vi "Configure Device.vi"(8 "error in":errorcluster, 11 "SR3XXX HVPS in":refnum<class "SR3XXX HVPS.lvclass">) -> (0 "error out":errorcluster, 3 "SR3XXX HVPS out":refnum<class "SR3XXX HVPS.lvclass">)   [LabVIEW 2014, in "SR3XXX HVPS.lvclass"]
uses:
  SR3XXX HVPS.lvclass
  <vilib>/Utility/config.llb/NI_LVConfig.lvlib
  reusable/Session APIs/File Access/Config Data/Config Data.lvclass
  <vilib>/Utility/config.llb/Read Key (String).vi
  <vilib>/Utility/config.llb/Read Key (Double).vi
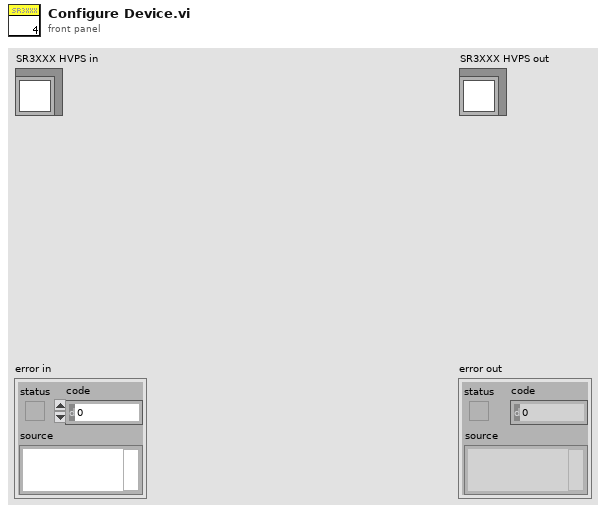
[diagram p1: front panel]
types:
  T1 = typedef "Config Data.lvclass/Config Session.ctl" = refnum<data-value>
  T2 = typedef "NI_LVConfig.lvlib/Config Data RefNum.ctl" = refnum<k1>
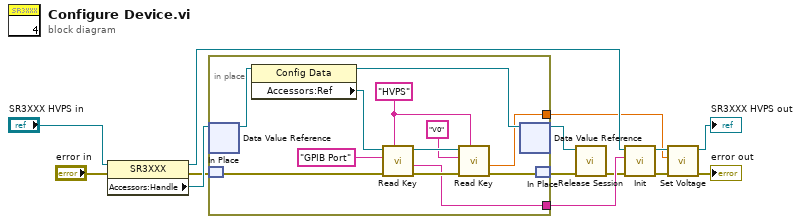
[diagram p0: block diagram]
diagram:
  n1 = property class="SR3XXX"(reference="SR3XXX HVPS in", error in="error in") -> (reference out=w9:refnum<class "SR3XXX HVPS.lvclass">, error out=w11:errorcluster, "Accessors:Handle"=w13:T1)
  n2 = in-place {
    in-place-border: [w16] -> w10
    in-place-border: [w15] -> w6
    w21 = "HVPS" ("section")
    n3 = in-place-dvr #1(w13) -> (w26:refnum<class "Config Data.lvclass">)  [unwired: 1 out]
    n4 = in-place-match #2(w11) -> (w18:errorcluster)
    n5 = property class="Config Data"(reference=w26) -> (reference out=w19:refnum<class "Config Data.lvclass">, "Accessors:Ref"=w25:T2)  [unwired: 1 in, 1 out]
    n6 = call-poly <vilib>:"Read Key.vi"("section"=w21, "error in (no error)"=w18, "key"="GPIB Port" ("section"), "refnum"=w25) -> ("error out"=w23:errorcluster, "value"=w16:string, "refnum out"=w22:T2)  [unwired: 4 in, 1 out]
    n7 = call-poly <vilib>:"Read Key.vi"("section"=w21, "error in (no error)"=w23, "key"="V0", "refnum"=w22) -> ("error out"=w17:errorcluster, "value"=w15:dbl)  [unwired: 4 in, 2 out]
    n8 = in-place-dvr #1(w19) -> (w3:T1)  [unwired: 1 out]
    n9 = in-place-match #2(w17) -> (w2:errorcluster)
  }
  n10 = call "Release Session.vi"("error in"=w2, "Session Handle"=w3) -> ("error out"=w1:errorcluster)  [unwired: 8 in, 1 out]
  n11 = call-dynamic "Init.vi"("error in"=w1, "Session"=w10, "SR3XXX HVPS in"=w9) -> ("error out"=w7:errorcluster, "SR3XXX HVPS out"=w8:refnum<class "SR3XXX HVPS.lvclass">)  [unwired: 7 in]
  n12 = call-dynamic "Set Voltage.vi"("error in (no error)"=w7, "V"=w6, "SR3XXX HVPS in"=w8) -> ("error out"=→"error out":errorcluster, "SR3XXX HVPS out"=→"SR3XXX HVPS out":refnum<class "SR3XXX HVPS.lvclass">)  [unwired: 7 in]
